vi "Get Max for Alarm.vi"(1 "Current Step Index":i32, 2 "Test Table":string[][](array[string]), 3 "Column Index for Max":i32=3) -> (0 "Min":dbl)   [LabVIEW 2018]
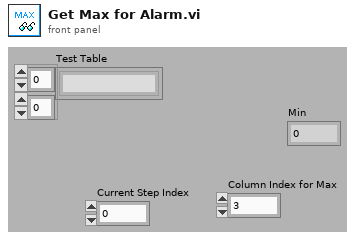
[diagram p1: front panel]
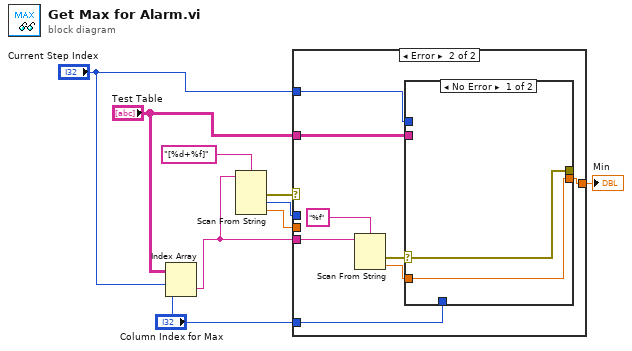
[diagram p0: block diagram]
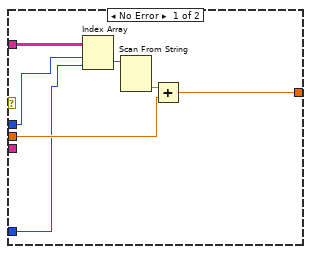
[diagram p2: hidden frame]
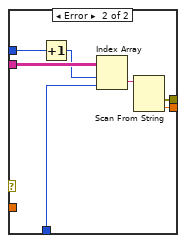
[diagram p3: hidden frame]
diagram:
  n1 = Index Array(array="Test Table", index (row)="Current Step Index", index (col)="Column Index for Max") -> (element=w2:string)
  n2 = Scan From String(format string="[%d+%f]", input string=w2) -> (error out=w5:errorcluster, output 1=w8:i32, output 2=w7:dbl)  [unwired: 4 in, 2 out]
  n3 = case shown="Error" w5 {
    tunnel: "Test Table" -> [w16 w21]
    tunnel: "Current Step Index" -> [_ w20]
    tunnel: w2 -> [_ w23]
    tunnel: w7 -> [w11 _]
    tunnel: [w12 w19] -> w9
    tunnel: w8 -> [w15 _]
    tunnel: "Column Index for Max" -> [w10 w17]
    frame No Error {
      n4 = Index Array(array=w16, index (row)=w15, index (col)=w10) -> (element=w14:string)
      n5 = Scan From String(input string=w14) -> (output 1=w13:dbl)  [unwired: 4 in, 3 out]
      n6 = Add(x=w13, y=w11) -> (x+y=w12:dbl)
    }
    frame Error {
      n7 = Scan From String(format string="%f", input string=w23) -> (error out=w22:errorcluster, output 1=w18:dbl)  [unwired: 3 in, 2 out]
      n8 = case shown="No Error" w22 {
        selector: w22 -> [w25 _]
        tunnel: w21 -> [_ w33]
        tunnel: w20 -> [_ w32]
        tunnel: [w26 w29] -> w19
        tunnel: w18 -> [w26 _]
        tunnel: w17 -> [_ w28]
        tunnel: [w25 w27] -> _
        frame No Error {
        }
        frame Error {
          n9 = Increment(x=w32) -> (x+1=w31:i32)
          n10 = Index Array(array=w33, index (row)=w31, index (col)=w28) -> (element=w30:string)
          n11 = Scan From String(input string=w30) -> (error out=w27:errorcluster, output 1=w29:dbl)  [unwired: 4 in, 2 out]
        }
      }
    }
  }
  "Min" <- w9
